vi "GetLedStates.vi"(8 "error in (no error)":errorcluster, 10 "ChainNumber":u8, 11 "ControlState in":T1 {"ChainMask" format="0x%02x"}) -> (0 "error out":errorcluster, 2 "LED Colors":u32[](array[colorbox]), 3 "ControlState out":T1 {"ChainMask" format="0x%02x"})   [LabVIEW 2023, in "ArduinoSerialBling.lvlib"]
uses:
  ArduinoSerialBling.lvlib
  ControlState.ctl
  ConnectionType.ctl
  UdpConnection.ctl
  ChainState.ctl
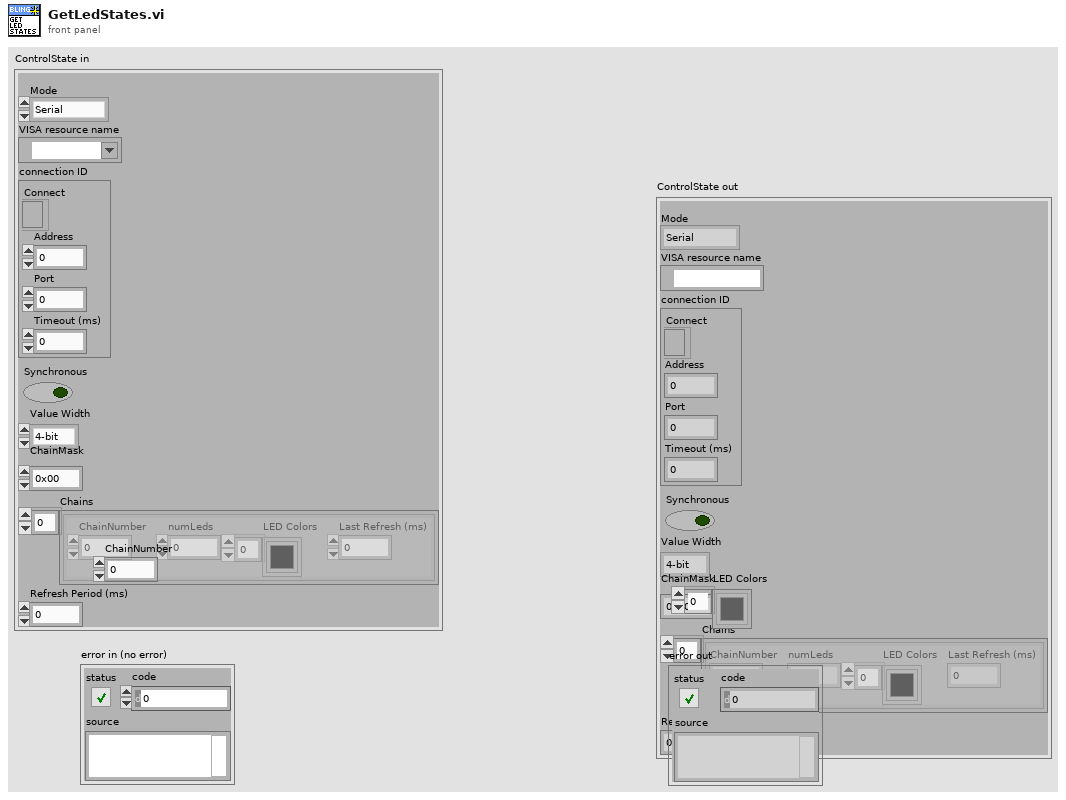
[diagram p1: front panel]
types:
  T1 = typedef "ArduinoSerialBling.lvlib/ControlState.ctl" = cluster{"Mode":T2, "VISA resource name":refnum<visa-resource-name>, "connection ID":T3, "Synchronous":bool, "Value Width":enum16{"4-bit", "8-bit"}, "ChainMask":u8, "Chains":T4[], "Refresh Period (ms)":u32}
  T2 = typedef "ConnectionType.ctl" = enum16{"Serial", "Ethernet", "Offline"}
  T3 = typedef "UdpConnection.ctl" = cluster{"Connect":refnum<k16>, "Address":u32, "Port":u16, "Timeout (ms)":i32}
  T4 = typedef "ArduinoSerialBling.lvlib/ChainState.ctl" = cluster{"ChainNumber":u8, "numLeds":u8, "LED Colors":u32[], "Last Refresh (ms)":u32}
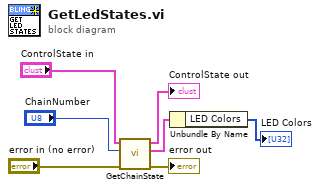
[diagram p0: block diagram]
diagram:
  n1 = call "GetChainState.vi"("error in (no error)"="error in (no error)", "ChainNumber"="ChainNumber", "ControlState in"="ControlState in") -> ("error out"=→"error out":errorcluster, "ChainState"=w2:T4, "ControlState out"=→"ControlState out":T1)  [unwired: 5 in, 1 out]
  n2 = Unbundle By Name(w2) -> ("LED Colors"=→"LED Colors":u32[])
